vi "Pack for gRPC.vi"(8 "error in":errorcluster, 9 "configuration / results":enum16{"Configuration", "Results"}(ring), 10 "data value":variant, 11 "measurement plugin in":refnum<class "FPT Pulse Measurement.lvclass">) -> (0 "error out":errorcluster, 2 "any":T1, 3 "measurement plugin out":refnum<class "FPT Pulse Measurement.lvclass">)   [LabVIEW 2023, in "FPT Pulse Measurement.lvclass"]
uses:
  FPT Pulse Measurement.lvclass
  <vilib>/gRPC/LabVIEW gRPC Library/Shared/Any.ctl
  Measurement Configuration.ctl
  Measurement Results.ctl
  2eca732d-dbaa-43bf-a7dd-ede2da65bc1b.vi
  a6012965-5700-4384-8228-972e71b6560c.vi
  <vilib>/gRPC/LabVIEW gRPC Library/Server API/Translate Protobuf Error.vi
  <vilib>/AdvancedString/1D String Array to Delimited String.vi
  <vilib>/gRPC/LabVIEW gRPC Library/Server API/Server/Get Server DLL Path.vi
  FPT Pulse Measurement.lvclass/FPT Pulse Measurement.ctl
  <vilib>/Plug-In SDKs/Measurements/Measurement Plugin Service/Measurement Plugin Service.lvclass
  <vilib>/gRPC/LabVIEW gRPC Library/grpc-lvsupport-release.lvlib
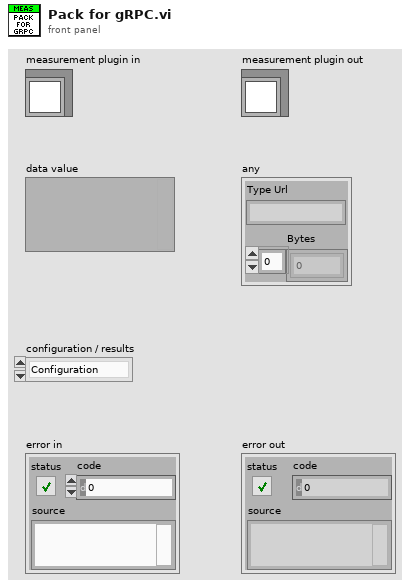
[diagram p1: front panel]
types:
  T1 = typedef "grpc-lvsupport-release.lvlib/Any.ctl" = cluster{"Type Url":string, "Bytes":u8[]}
  T2 = typedef "grpc-lvsupport-release.lvlib/grpcId.ctl" = u64
  T3 = typedef "FPT Pulse Measurement.lvclass/Measurement Configuration.ctl" = cluster{"Automation Test":bool, "Power sequencing file path":string, "RFSG name":string, "RFSG port":string, "RFSG attenuation mode":enum32{"<None>", "Constant Attenuation", "s2p File"}, "RFSG external attenuation (dB)":dbl, "RFSG s-parameters orientation":enum32{"Port1 Towards DUT", "Port2 Towards DUT"}, "RFSG s2p file path":string, "RFmx name":string, "RFmx port":string, "RFmx attenuation mode":enum32{"<None>", "Constant Attenuation", "s2p File"}, "RFmx external attenuation (dB)":dbl, "RFmx s-parameters orientation":enum32{"Port1 Towards DUT", "Port2 Towards DUT"}, "RFmx s2p file path":string, "RFmx Center Frequency (Hz)":dbl, "RFmx Measurement Bandwidth (Hz)":dbl, "RFmx Reference Level (dBm)":dbl, "RFSG Generation IQ Rate (S/s)":dbl, "Pulse Acquisition Length (s)":dbl, "Pulse Power Level (dBm)":dbl, "Pulse Repetition Interval [PRI] (s)":dbl, "Pulse Width (s)":dbl, "Number of Pulses per Burst":u32, "Measurement Offset":i32, "Window Start (%)":dbl, "Window Stop (%)":dbl, "Window Step Size (%)":dbl, "High Reference Level (%)":dbl, "Width Reference Level (%)":dbl, "Low Reference Level (%)":dbl}
  T4 = typedef "FPT Pulse Measurement.lvclass/Measurement Results.ctl" = cluster{"Status":string, "TS Intrapulse Stability":dbl[][], "TS P2P Stability":dbl[][], "Per Pulse Result":dbl[][], "Per Pulse Result (Name)":string[], "Duty Cycle (%)":dbl, "Rising Time (us)":dbl, "Fall Time (us)":dbl, "Droop (%)":dbl, "Ripple (%)":dbl, "Overshoot (%)":dbl, "Amplitude Stability (dB)":dbl, "Phase Stability (dB)":dbl}
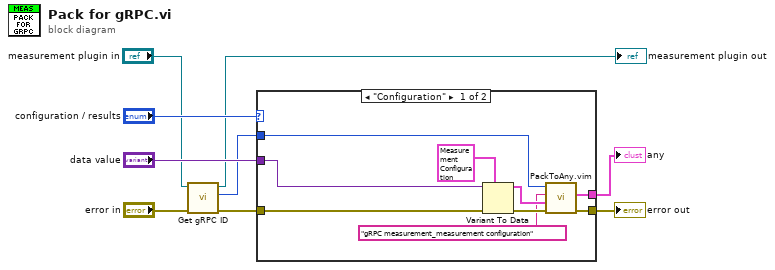
[diagram p0: block diagram]
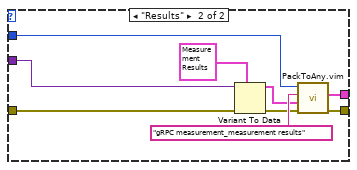
[diagram p2: hidden frame]
diagram:
  n1 = call <vilib>:"Get gRPC ID.vi"("error in"="error in", "measurement plugin service in"="measurement plugin in") -> ("error out"=w4:errorcluster, "gRPC ID"=w1:T2, "measurement plugin service out"=→"measurement plugin out":refnum<class "FPT Pulse Measurement.lvclass">)  [unwired: 7 in]
  n2 = case shown="\"Configuration\"" "configuration / results" {
    tunnel: w4 -> [w18 w27]
    tunnel: "data value" -> [w17 w26]
    tunnel: w1 -> [w14 w22]
    tunnel: [w16 w24] -> w8
    tunnel: [w15 w23] -> w7
    frame "Configuration" {
      n3 = Variant To Data(error in=w18, type=T3 {"Automation Test"=FALSE, "Power sequencing file path"="Lorem ipsum dolor sit", "RFSG name"="5842_0", "RFSG port"="", "RFSG attenuation mode"=enum."s2p File", "RFSG external attenuation (dB)"=64.0, "RFSG s-parameters orientation"=enum."Port1 Towards DUT", "RFSG s2p file path"="", "RFmx name"="Lorem ipsum dolor sit", "RFmx port"="", "RFmx attenuation mode"=enum."Constant Attenuation", "RFmx external attenuation (dB)"=-64.0, "RFmx s-parameters orientation"=enum."Port2 Towards DUT", "RFmx s2p file path"="", "RFmx Center Frequency (Hz)"=10000000000.0, "RFmx Measurement Bandwidth (Hz)"=80000000.0, "RFmx Reference Level (dBm)"=10.0, "RFSG Generation IQ Rate (S/s)"=10000000000.0, "Pulse Acquisition Length (s)"=80000000.0, "Pulse Power Level (dBm)"=10.0, "Pulse Repetition Interval [PRI] (s)"=1250000000.0, "Pulse Width (s)"=0.001, "Number of Pulses per Burst"=0, "Measurement Offset"=0, "Window Start (%)"=2e-05, "Window Stop (%)"=20.0, "Window Step Size (%)"=0.0, "High Reference Level (%)"=10.0, "Width Reference Level (%)"=90.0, "Low Reference Level (%)"=10.0} ("measurement configuration"), Variant=w17) -> (data=w13:T3, error out=w12:errorcluster)
      n4 = call "PackToAny.vim"("error in"=w12, "Data To Pack"=w13, "Message Type"="gRPC measurement_measurement configuration", "gRPCid in"=w14) -> ("error out"=w16:errorcluster, "Any"=w15:T1)  [unwired: 5 in, 1 out]
    }
    frame "Results" {
      n5 = Variant To Data(error in=w27, type=T4 {"Status"="Empty", "TS Intrapulse Stability"=[], "TS P2P Stability"=[], "Per Pulse Result"=[], "Per Pulse Result (Name)"=[], "Duty Cycle (%)"=0.0, "Rising Time (us)"=0.0, "Fall Time (us)"=0.0, "Droop (%)"=0.0, "Ripple (%)"=0.0, "Overshoot (%)"=0.0, "Amplitude Stability (dB)"=0.0, "Phase Stability (dB)"=0.0} ("Measurement Results"), Variant=w26) -> (data=w20:T4, error out=w19:errorcluster)
      n6 = call "PackToAny.vim"("error in"=w19, "Data To Pack"=w20, "Message Type"="gRPC measurement_measurement results", "gRPCid in"=w22) -> ("error out"=w24:errorcluster, "Any"=w23:T1)  [unwired: 5 in, 1 out]
    }
  }
  "error out" <- w8
  "any" <- w7
